vi "LSI218Data_measure.vi"(0 "LSI218Data in":refnum<class "LSI218Data.lvclass">, 5 "MeasurementIndex":i32, 11 "error in (no error)":errorcluster) -> (1 "TimeMeasuremeent":timestamp, 3 "Active?":bool[](array[boolean]), 4 "LSI218Data out":refnum<class "LSI218Data.lvclass">, 6 "LastMeasurementConfig":T1(array[cluster]), 8 "LastData":dbl[](array[numeric]), 10 "Status":u16(ring)=2 items=["Initialized", "Ready", "Measuring", "Terminated"], 12 "TimeArray":timestamp[](array[timestamp]), 13 "DataArray":dbl[][](array[numeric]), 15 "error out":errorcluster)   [LabVIEW 2017, in "LSI218Data.lvclass"]
uses:
  LSI218Data.lvclass
  LSI218Data.lvclass/LSI218Data.ctl
  istr.lib/Lake Shore Cryotronics 218/Lake Shore Cryotronics 218.lvlib
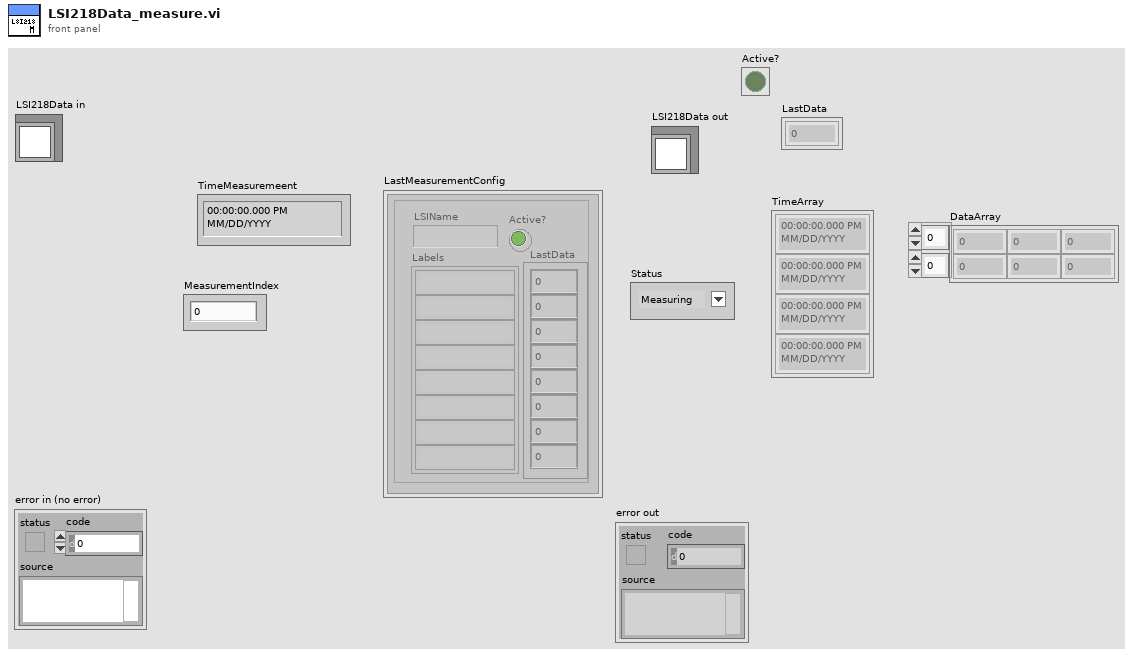
[diagram p1: front panel]
types:
  T1 = cluster{"LSIName":string, "Active?":bool, "LastData":dbl[], "Labels":string[]}[]
  T2 = enum16{"Initialized", "Ready", "Measuring", "Terminated"}
  T3 = cluster{"LSIName":string, "Labels":string[], "SensorLocations":enum16{"N.C.", "T3He1-1", "T3He1-2", "T3He1-3", "T3He1-4", "T3He2-1", "T3He2-2", "T3He3", "T3He4", "T3He5", "T3He6-1", "T3He6-2", "T3He7-1", "T3He7-2", "T3He8", "T3He9", "T3He10", "T4He1", "T4He2-1", "T4He2-2", "T4He3-1", "T4He3-2", "T4He3-3", "T4He3-4", "T4He4", "T4He5", "T4He6", "T4He7", "T4He8", "T4He9", "T4He10", "T1K1", "T1K2", "T1K3-1", "T1K3-2", "T1K4", "T1K5", "T1K6", "TIP1", "TIP2", "TIP3", "TIP4", "TIP5", "TIP6", "TIP7", "TTH1", "TTH2", "TTH3", "TTH4"}[], "Active?":bool, "VISA res. name":refnum<visa-resource-name>}[]
  T4 = cluster{"LSIName":string, "Labels":string[], "SensorLocations":enum16{"N.C.", "T3He1-1", "T3He1-2", "T3He1-3", "T3He1-4", "T3He2-1", "T3He2-2", "T3He3", "T3He4", "T3He5", "T3He6-1", "T3He6-2", "T3He7-1", "T3He7-2", "T3He8", "T3He9", "T3He10", "T4He1", "T4He2-1", "T4He2-2", "T4He3-1", "T4He3-2", "T4He3-3", "T4He3-4", "T4He4", "T4He5", "T4He6", "T4He7", "T4He8", "T4He9", "T4He10", "T1K1", "T1K2", "T1K3-1", "T1K3-2", "T1K4", "T1K5", "T1K6", "TIP1", "TIP2", "TIP3", "TIP4", "TIP5", "TIP6", "TIP7", "TTH1", "TTH2", "TTH3", "TTH4"}[], "Active?":bool, "VISA res. name":refnum<visa-resource-name>}
  T5 = cluster{"LSIName":string, "Active?":bool, dbl[], "Labels":string[]}
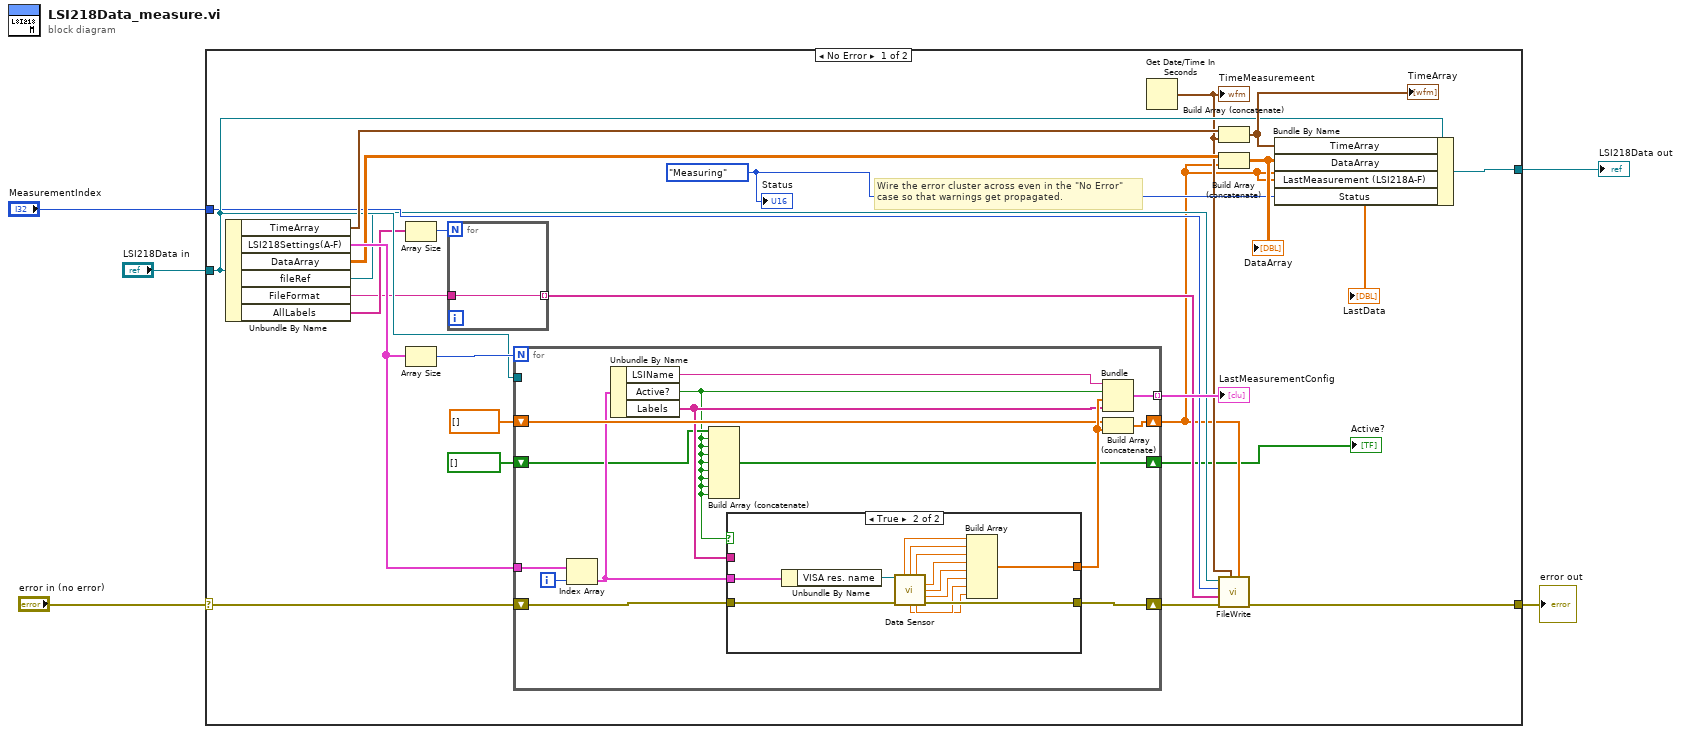
[diagram p0: block diagram]
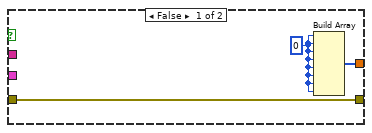
[diagram p2: hidden frame]
diagram:
  n1 = case shown="No Error" "error in (no error)" {
    selector: "error in (no error)" -> [w22 w61]
    tunnel: [w29 w62] -> w3
    tunnel: "LSI218Data in" -> [w19 w62]
    tunnel: [w10 w61] -> w2
    tunnel: "MeasurementIndex" -> [w15 _]
    frame No Error {
      w20 = T2."Measuring" ("Status")
      # "Wire the error cluster across even in the \"No Error\"\ncase so that warnings get propagated."
      n2 = Unbundle By Name(w19) -> ("TimeArray"=w28:timestamp[], "LSI218Settings(A-F)"=w25:T3, "DataArray"=w24:dbl[][], "fileRef"=w13:refnum<file>, "FileFormat"=w16:string, "AllLabels"=w18:string[])
      n3 = Array Size(array=w18) -> (size(s)=w17:i32)
      n4 = Array Size(array=w25) -> (size(s)=w26:i32)
      n5 = for {
        N: w17 -> [_]
        tunnel: [w30] -> w14 mode=indexing
        tunnel: w16 -> [w30]
      }
      n6 = for {
        N: w26 -> [_]
        tunnel: w25 -> [w44]
        tunnel: w19 -> [_]
        tunnel: [w42] -> w21 mode=indexing
        shift-right: [w40] -> w9
        shift-left: dbl[] [] -> [w39]
        shift-right: [w36] -> w11
        shift-left: w22 -> [w35]
        shift-right: [w33] -> w6
        shift-left: bool[] [] -> [w32]
        i -> [w38]
        n7 = Index Array(array=w44, index=w38) -> (element=w37:T4)
        n8 = Unbundle By Name(w37) -> ("LSIName"=w43:string, "Active?"=w31:bool, "Labels"=w34:string[])
        n9 = Build Array (concatenate)(w32, w31, w31, w31, w31, w31, w31, w31, w31) -> (w33:bool[])
        n10 = case shown="True" w31 {
          tunnel: [w46 w56] -> w41
          tunnel: w37 -> [_ w60]
          tunnel: [w45 w58] -> w36
          tunnel: w35 -> [w45 w57]
          tunnel: w34 -> [_ _]
          frame False {
            w47 = 0
            n11 = Build Array(w47, w47, w47, w47, w47, w47, w47, w47) -> (w46:i32[])
          }
          frame True {
            n12 = Unbundle By Name(w60) -> ("VISA res. name"=w59:refnum<visa-resource-name>)
            n13 = call "Data Sensor.vi"("VISA resource name"=w59, "error in (no error)"=w57) -> ("Input 1"=w55:dbl, "Input 2"=w54:dbl, "Input 3"=w53:dbl, "Input 4"=w52:dbl, "Input 5"=w51:dbl, "Input 6"=w50:dbl, "Input 8"=w48:dbl, "Input 7"=w49:dbl, "error out"=w58:errorcluster)  [unwired: 4 in, 1 out]
            n14 = Build Array(w55, w54, w53, w52, w51, w50, w49, w48) -> (w56:dbl[])
          }
        }
        n15 = Bundle("LSIName"=w43, "Active?"=w31, w41, "Labels"=w34) -> (w42:T5)  [unwired: 1 in]
        n16 = Build Array (concatenate)(w39, w41) -> (w40:dbl[])
      }
      "LastMeasurementConfig" <- w21
      "Active?" <- w6
      "LastData" <- w9
      n17 = Get Date/Time In Seconds() -> (seconds since 1Jan1904=w12:timestamp)
      "TimeMeasuremeent" <- w12
      n18 = Build Array (concatenate)(w28, w12) -> (w27:timestamp[])
      "TimeArray" <- w27
      n19 = Build Array (concatenate)(w24, w9) -> (w23:dbl[][])
      "DataArray" <- w23
      n20 = call "FileWrite.vi"("DataArray"=w9, "Time Stamp"=w12, "Error In"=w11, "FileFormat"=w14, "Index"=w15, "refnum in"=w13) -> ("Error Out"=w10:errorcluster)  [unwired: 4 in, 1 out]
      n21 = Bundle By Name(cluster=w19, "TimeArray"=w27, "DataArray"=w23, "LastMeasurement (LSI218A-F)"=w9, "Status"=w20) -> (w29:refnum<class "LSI218Data.lvclass">)
      "Status" <- w20
    }
    frame Error {
    }
  }
  "error out" <- w2
  "LSI218Data out" <- w3
